vi "Sample Pad Example.vi"() -> ()   [LabVIEW 2020]
doc: "A simple sample pad, which can trigger up to 16 simultaneous sound effects. Demonstrates the Mixer component, including file loading, playback, and mixer audio monitoring via a music visualizer."
uses:
  Mixer/Channel/Controls/Channel State.ctl
  Mixer/Mixer/Mixer.lvclass/Mixer.ctl
  e8fa8eb6-c38c-4b8a-b362-922d187964a0.vi
  Mixer/Mixer/Polymorphic VIs/Channel Load (Path).vi
  Mixer/Mixer/Mixer.lvclass
  Mixer/Channel/Channel.lvclass
panel:
  in  "Labels Checkbox":bool=TRUE
  in  "Visualizer":bool
  in  "Sample Path":path
  in  "Stop":bool
  in  "Play 4":bool caption="V"
  in  "Play 3":bool caption="C"
  in  "Play 2":bool caption="X"
  in  "Play 1":bool caption="Z"
  in  "Play 8":bool caption="F"
  in  "Play 7":bool caption="D"
  in  "Play 6":bool caption="S"
  in  "Play 5":bool caption="A"
  in  "Play 12":bool caption="R"
  in  "Play 11":bool caption="E"
  in  "Play 10":bool caption="W"
  in  "Play 9":bool caption="Q"
  in  "Play 16":bool caption="4"
  in  "Play 15":bool caption="3"
  in  "Play 14":bool caption="2"
  in  "Play 13":bool caption="1"
  # "Instructions:\n1. Run the VI.\n2. Select a Sample Path which contains multiple audio files.\n3. Click a button or press the corresponding keyboard key to\n    play the audio sample.\n4. Samples can be played simultaneously, or retriggered by\n    pressing the same button / key in quick succession."
  # "G"
  # "-Audio"
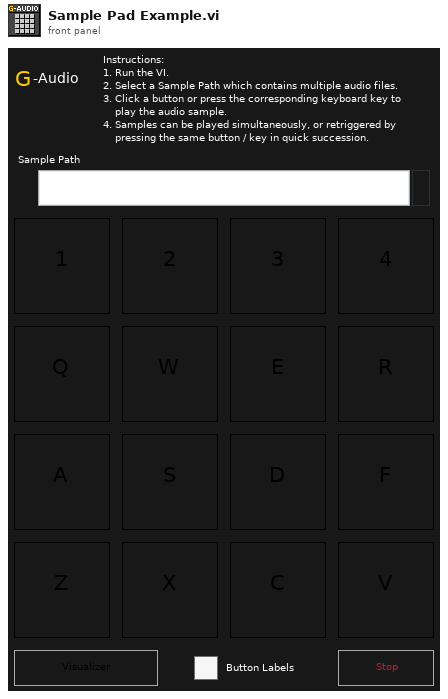
[diagram p1: front panel]
types:
  T1 = typedef "G-Audio.lvlib/Channel.lvclass/Channel State.ctl" = enum16{"Empty", "Error", "Loading", "Loaded", "Stopped", "Paused", "Playing", "Retrigger"}
  T2 = enum32{"Invalid", "Standard", "Closed", "Hidden", "Minimized", "Maximized"}
  T3 = typedef "G-Audio.lvlib/Channel.lvclass/Channel Status.ctl" = cluster{"Frame":u64, "State":T1, "Volume":dbl}
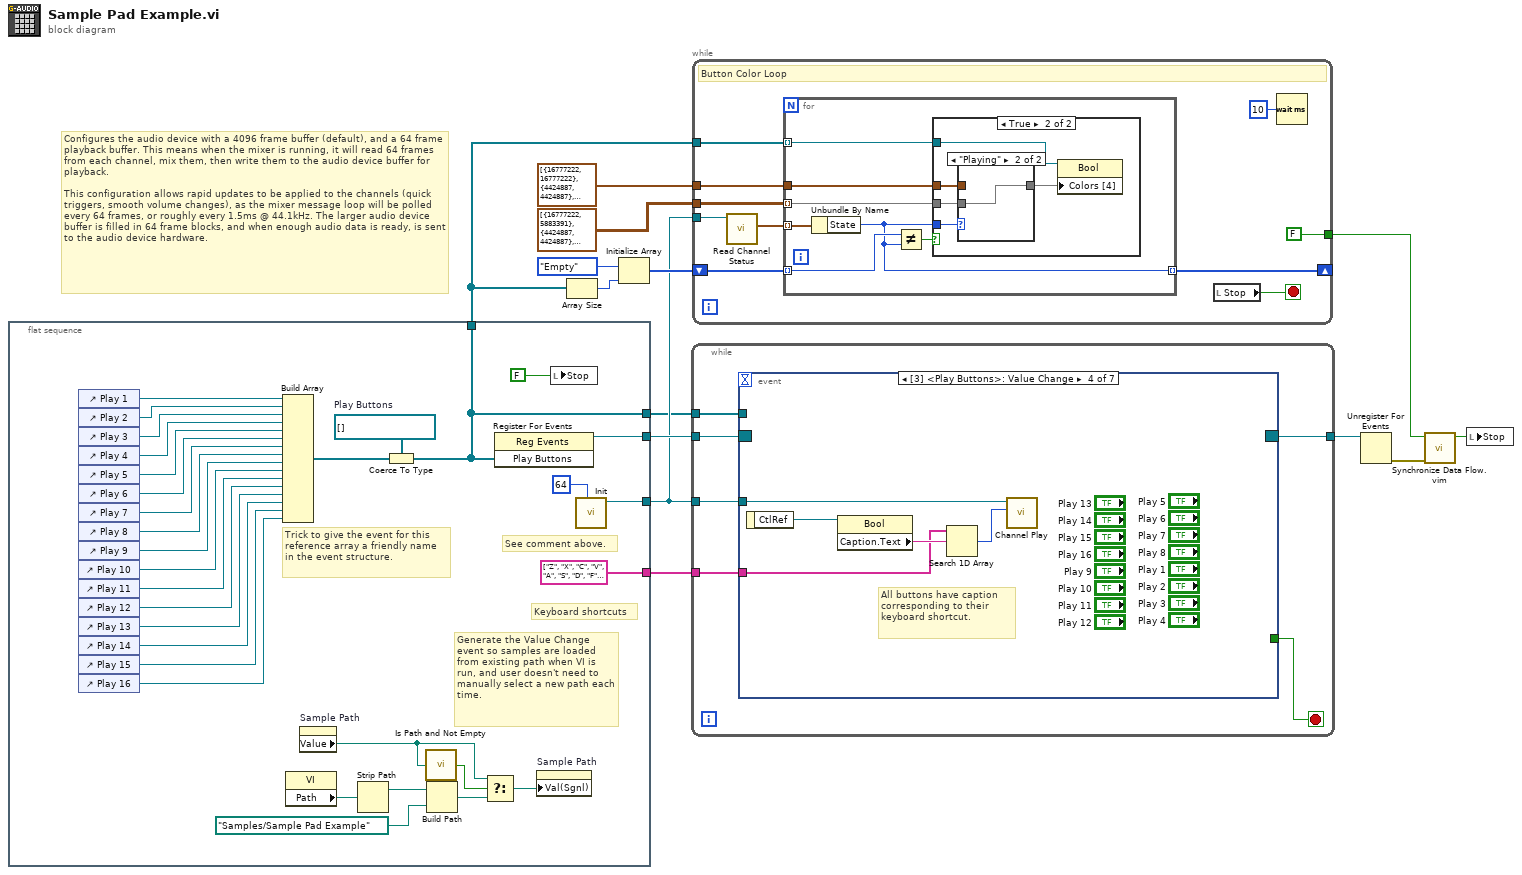
[diagram p0: block diagram]
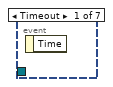
[diagram p4: hidden frame]
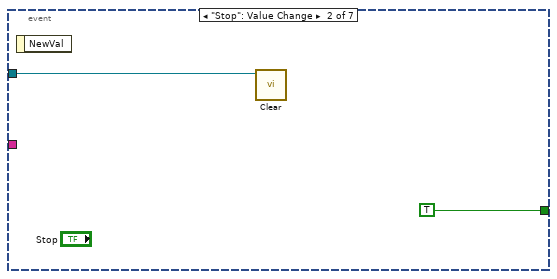
[diagram p5: hidden frame]
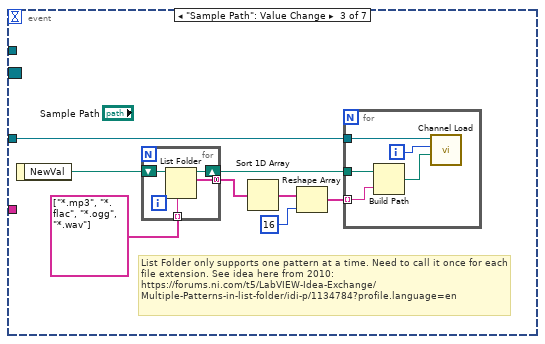
[diagram p6: hidden frame]
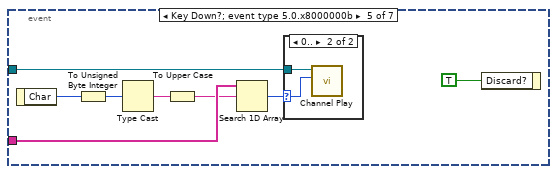
[diagram p7: hidden frame]
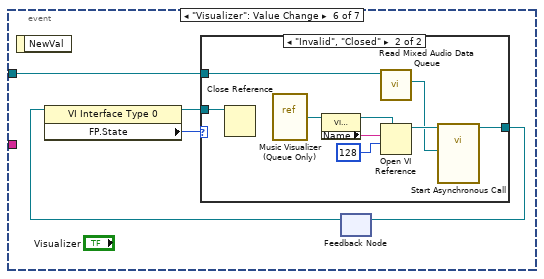
[diagram p9: hidden frame]
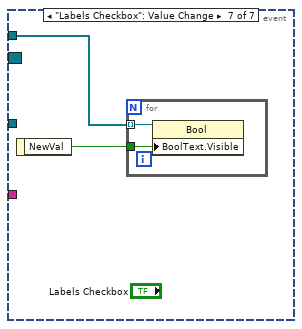
[diagram p11: hidden frame]
diagram:
  # "Configures the audio device with a 4096 frame buffer (default), and a 64 frame playback buffer. This means when the mixer is running, it will read 64 frames from each channel, mix them, then write them to the audio device buffer for playback.\n\nThis configuration allows rapid updates to be applied to the channels (quick triggers, smooth volume changes), as the mixer message loop will be polled every 64 frames, or roughly every 1.5ms @ 44.1kHz. The larger audio device buffer is filled in 64 frame blocks, and when enough audio data is ready, is sent to the audio device hardware."
  n1 = flat-sequence {
    tunnel: [w44] -> w13
    tunnel: [string[] ["Z", "X", "C", "V", "A", "S", "D", "F", "Q", "W", "E", "R", "1", "2", "3", "4"]] -> w12
    tunnel: [w15] -> w2
    tunnel: [w42] -> w5
    tunnel: [w15] -> w1
    frame #0 {
      w45 = refnum<vi>[] []  # Play Buttons
      # "Trick to give the event for this reference array a friendly name in the event structure."
      # "See comment above."
      # "Generate the Value Change event so samples are loaded from existing path when VI is run, and user doesn't need to manually select a new path each time."
      # "Keyboard shortcuts"
      n2 = control-ref of="Play 1"() -> (w39:refnum<vi>)
      n3 = control-ref of="Play 2"() -> (w38:refnum<vi>)
      n4 = control-ref of="Play 3"() -> (w37:refnum<vi>)
      n5 = control-ref of="Play 4"() -> (w36:refnum<vi>)
      n6 = control-ref of="Play 5"() -> (w35:refnum<vi>)
      n7 = control-ref of="Play 6"() -> (w34:refnum<vi>)
      n8 = control-ref of="Play 7"() -> (w33:refnum<vi>)
      n9 = control-ref of="Play 8"() -> (w32:refnum<vi>)
      n10 = control-ref of="Play 9"() -> (w31:refnum<vi>)
      n11 = control-ref of="Play 10"() -> (w30:refnum<vi>)
      n12 = control-ref of="Play 11"() -> (w29:refnum<vi>)
      n13 = control-ref of="Play 12"() -> (w28:refnum<vi>)
      n14 = control-ref of="Play 13"() -> (w27:refnum<vi>)
      n15 = control-ref of="Play 14"() -> (w26:refnum<vi>)
      n16 = control-ref of="Play 15"() -> (w25:refnum<vi>)
      n17 = control-ref of="Play 16"() -> (w24:refnum<vi>)
      n18 = Build Array(w39, w38, w37, w36, w35, w34, w33, w32, w31, w30, w29, w28, w27, w26, w25, w24) -> (w40:refnum<vi>[])
      n19 = property class="VI"() -> ("Path"=w21:path)  [unwired: 2 in, 2 out]
      n20 = property on="Sample Path" class="Path"() -> ("Value"=w17:path)  [unwired: 2 in, 2 out]
      n21 = Strip Path(path=w21) -> (stripped path=w20:path)  [unwired: 1 out]
      n22 = Coerce To Type(0:w40, 1:w45) -> (2:w15:refnum<vi>[])
      n23 = call <vilib>:"Is Path and Not Empty.vi"("path"=w17) -> ("Is Path and Not Empty?"=w23:bool)  [unwired: 4 in]
      n24 = Build Path(base path=w20, name or relative path=path "Samples/Sample Pad Example") -> (appended path=w18:path)
      n25 = Select(t=w17, s=w23, f=w18) -> (s? t:f=w22:path)
      n26 = register-events(w15) -> (reference out=w44:refnum<event-registration>)  [unwired: 2 in, 1 out]
      n27 = property on="Sample Path" class="Path"("Val(Sgnl)"=w22) -> ()  [unwired: 2 in, 2 out]
      n28 = local write "Stop"(FALSE ("Stop")) -> ()
      n29 = call "Init.vi"("Playback Size (4096)"=64) -> ("Mixer out"=w42:refnum<class "Mixer.lvclass">)  [unwired: 9 in, 1 out]
    }
  }
  n30 = Array Size(array=w2) -> (size(s)=w3:i32)
  n31 = Initialize Array(Channel_State."Empty" ("State"), w3) -> (w14:T1[])
  n32 = while {
    tunnel: w13 -> [w51]
    tunnel: w5 -> [w50]
    tunnel: w12 -> [w49]
    tunnel: [w47] -> w11
    tunnel: w1 -> [w46]
    stop <- w48 stop-if-true
    n33 = event shown="[3] <Play Buttons>: Value Change" {
      selector: w51 -> [_ _ _ _ _ _ _]
      dyn-events: [_ _ _ _ _ _ _] -> w47
      timeout: _ -> [_ _ _ _ _ _ _]
      tunnel: w50 -> [_ w53 w59 w74 w83 w89 _]
      tunnel: w49 -> [_ _ _ w72 w81 _ _]
      tunnel: [_ TRUE _ _ _ _ _] -> w48
      tunnel: w46 -> [_ _ _ _ _ _ w102]
      event Timeout {
        n34 = event-data() -> ()  [unwired: 1 in, 1 out]
      }
      event "Stop": Value Change {
        n35 = event-data() -> ()  [unwired: 1 in, 1 out]
        n36 = call "Clear.vi"("Mixer in"=w53) -> ()  [unwired: 10 in, 1 out]
      }
      event "Sample Path": Value Change {
        # "List Folder only supports one pattern at a time. Need to call it once for each file extension. See idea here from 2010:\nhttps://forums.ni.com/t5/LabVIEW-Idea-Exchange/Multiple-Patterns-in-list-folder/idi-p/1134784?profile.language=en"
        n37 = event-data() -> ("NewVal"=w54:path)  [unwired: 1 in]
        n38 = for {
          shift-right: [w65] -> w60
          shift-left: w54 -> [w64]
          tunnel: string[] ["*.mp3", "*.flac", "*.ogg", "*.wav"] -> [w63] mode=indexing
          tunnel: [w62] -> w56 mode=concatenating
          n39 = List Folder(path=w64, pattern=w63) -> (path out=w65:path, filenames=w62:string[])  [unwired: 2 in, 2 out]
        }
        n40 = Sort 1D Array(array=w56) -> (sorted array=w55:string[])
        n41 = Reshape Array(w55, 16 ("dimension size")) -> (w61:string[])
        n42 = for {
          tunnel: w61 -> [w70] mode=indexing
          tunnel: w60 -> [w69]
          tunnel: w59 -> [w68]
          i -> [w67]
          n43 = Build Path(base path=w69, name or relative path=w70) -> (appended path=w66:path)
          n44 = call-poly "Channel Load.vi"("Path"=w66, "Channel Index"=w67, "Mixer in"=w68) -> ()  [unwired: 7 in, 2 out]
        }
      }
      event Value Change {
        # "All buttons have caption corresponding to their keyboard shortcut."
        n45 = event-data() -> ("CtlRef"=w75:refnum<vi>)  [unwired: 1 in]
        n46 = property class="Bool"(reference=w75) -> ("Caption.Text"=w73:string)  [unwired: 1 in, 2 out]
        n47 = Search 1D Array(1D array=w72, element=w73) -> (index of element=w71:i32)  [unwired: 1 in]
        n48 = call "Channel Play.vi"("Channel Index"=w71, "Mixer in"=w74) -> ()  [unwired: 8 in, 2 out]
      }
      event Key Down?; event type 5.0.x8000000b {
        n49 = event-data() -> ("Char"=w82:i16)  [unwired: 1 in]
        n50 = To Unsigned Byte Integer(number=w82) -> (unsigned 8bit integer=w78:u8)
        n51 = Type Cast(x=w78) -> (*(type *) &x=w76:string)  [unwired: 1 in]
        n52 = To Upper Case(1:w76) -> (0:w79:string)
        n53 = Search 1D Array(1D array=w81, element=w79) -> (index of element=w77:i32)  [unwired: 1 in]
        n54 = case shown="0.." w77 {
          selector: w77 -> [_ w84]
          tunnel: w83 -> [_ w85]
          frame Default {
          }
          frame 0.. {
            n55 = call "Channel Play.vi"("Channel Index"=w84, "Mixer in"=w85) -> ()  [unwired: 8 in, 2 out]
          }
        }
        n56 = event-data("Discard?"=TRUE) -> ()  [unwired: 1 in, 1 out]
      }
      event "Visualizer": Value Change {
        n57 = event-data() -> ()  [unwired: 1 in, 1 out]
        n58 = feedback #1() -> (w86:refnum<vi>)  [unwired: 1 in]
        n59 = property class="VI Interface Type 0"(reference=w86) -> (reference out=w88:refnum<vi>, "FP.State"=w87:T2)  [unwired: 1 in, 1 out]
        n60 = case shown="\"Invalid\", \"Closed\"" w87 {
          tunnel: [w91 w95] -> w90
          tunnel: w89 -> [_ w94]
          tunnel: w88 -> [w91 w92]
          frame Default {
          }
          frame "Invalid", "Closed" {
            n61 = Close Reference(reference=w92) -> ()  [unwired: 1 in, 1 out]
            n62 = vi-ref "Music Visualizer (Queue Only).vi"() -> (w100:refnum<vi>)
            n63 = property class="VI (strict)"(reference=w100) -> (reference out=w98:refnum<vi>, "Name"=w99:string)  [unwired: 1 in, 1 out]
            n64 = call "Read Mixed Audio Data Queue.vi"("Mixer in"=w94) -> ("Mixed Audio Data"=w93:refnum<queue>)  [unwired: 8 in, 2 out]
            n65 = Open VI Reference(type specifier VI Refnum (for type only)=w98, vi path=w99, options=128) -> (vi reference=w96:refnum<vi>)  [unwired: 3 in, 1 out]
            n66 = call-by-ref "Start Asynchronous Call"(reference=w96, "Mixed Audio Data"=w93) -> (reference out=w95:refnum<vi>)  [unwired: 12 in, 1 out]
          }
        }
        n67 = feedback-in #1(w90) -> ()
      }
      event "Labels Checkbox": Value Change {
        n68 = event-data() -> ("NewVal"=w101:bool)  [unwired: 1 in]
        n69 = for {
          tunnel: w102 -> [w104] mode=indexing
          tunnel: w101 -> [w103]
          n70 = property class="Bool"(reference=w104, "BoolText.Visible"=w103) -> ()  [unwired: 1 in, 2 out]
        }
      }
    }
  }
  n71 = while {
    tunnel: w5 -> [w114]
    tunnel: w2 -> [w112]
    tunnel: cluster{u32, u32}[] [{16777222, 16777222}, {4424887, 4424887}, {4424887, 4424887}, {4424887, 4424887}] ("Colors [4]") -> [w111]
    tunnel: cluster{"Color Box":u32, "Color Box":u32}[][] [[{"Color Box"=16777222, "Color Box"=5883391}, {"Color Box"=4424887, "Color Box"=4424887}, {"Color Box"=4424887, "Color Box"=4424887}, {"Color Box"=4424887, "Color Box"=4424887}], [{"Color Box"=16777222, "Color Box"=5883391}, {"Color Box"=4424887, "Color Box"=4424887}, {"Color Box"=4424887, "Color Box"=4424887}, {"Color Box"=4424887, "Color Box"=4424887}], [{"Color Box"=16777222, "Color Box"=5883391}, {"Color Box"=4424887, "Color Box"=4424887}, {"Color Box"=4424887, "Color Box"=4424887}, {"Color Box"=4424887, "Color Box"=4424887}], [{"Color Box"=16777222, "Color Box"=5883391}, {"Color Box"=4424887, "Color Box"=4424887}, {"Color Box"=4424887, "Color Box"=4424887}, {"Color Box"=4424887, "Color Box"=4424887}], [{"Color Box"=16777222, "Color Box"=6618880}, {"Color Box"=4424887, "Color Box"=4424887}, {"Color Box"=4424887, "Color Box"=4424887}, {"Color Box"=4424887, "Color Box"=4424887}], [{"Color Box"=16777222, "Color Box"=6618880}, {"Color Box"=4424887, "Color Box"=4424887}, {"Color Box"=4424887, "Color Box"=4424887}, {"Color Box"=4424887, "Color Box"=4424887}], [{"Color Box"=16777222, "Color Box"=6618880}, {"Color Box"=4424887, "Color Box"=4424887}, {"Color Box"=4424887, "Color Box"=4424887}, {"Color Box"=4424887, "Color Box"=4424887}], [{"Color Box"=16777222, "Color Box"=6618880}, {"Color Box"=4424887, "Color Box"=4424887}, {"Color Box"=4424887, "Color Box"=4424887}, {"Color Box"=4424887, "Color Box"=4424887}], [{"Color Box"=16777222, "Color Box"=16746514}, {"Color Box"=4424887, "Color Box"=4424887}, {"Color Box"=4424887, "Color Box"=4424887}, {"Color Box"=4424887, "Color Box"=4424887}], [{"Color Box"=16777222, "Color Box"=16746514}, {"Color Box"=4424887, "Color Box"=4424887}, {"Color Box"=4424887, "Color Box"=4424887}, {"Color Box"=4424887, "Color Box"=4424887}], [{"Color Box"=16777222, "Color Box"=16746514}, {"Color Box"=4424887, "Color Box"=4424887}, {"Color Box"=4424887, "Color Box"=4424887}, {"Color Box"=4424887, "Color Box"=4424887}], [{"Color Box"=16777222, "Color Box"=16746514}, {"Color Box"=4424887, "Color Box"=4424887}, {"Color Box"=4424887, "Color Box"=4424887}, {"Color Box"=4424887, "Color Box"=4424887}], [{"Color Box"=16777222, "Color Box"=16711680}, {"Color Box"=4424887, "Color Box"=4424887}, {"Color Box"=4424887, "Color Box"=4424887}, {"Color Box"=4424887, "Color Box"=4424887}], [{"Color Box"=16777222, "Color Box"=16711680}, {"Color Box"=4424887, "Color Box"=4424887}, {"Color Box"=4424887, "Color Box"=4424887}, {"Color Box"=4424887, "Color Box"=4424887}], [{"Color Box"=16777222, "Color Box"=16711680}, {"Color Box"=4424887, "Color Box"=4424887}, {"Color Box"=4424887, "Color Box"=4424887}, {"Color Box"=4424887, "Color Box"=4424887}], [{"Color Box"=16777222, "Color Box"=16711680}, {"Color Box"=4424887, "Color Box"=4424887}, {"Color Box"=4424887, "Color Box"=4424887}, {"Color Box"=4424887, "Color Box"=4424887}]] ("appended array") -> [w110]
    tunnel: [FALSE ("Stop")] -> w7
    shift-right: [w106] -> _
    shift-left: w14 -> [w105]
    stop <- w108 stop-if-true
    # "Button Color Loop"
    n72 = call "Read Channel Status.vi"("Mixer in"=w114) -> ("Channel Status"=w113:T3[])  [unwired: 8 in, 2 out]
    n73 = for {
      tunnel: w113 -> [w121] mode=indexing
      tunnel: w112 -> [w120] mode=indexing
      tunnel: w111 -> [w119]
      tunnel: w110 -> [w118] mode=indexing
      tunnel: [w115] -> w106 mode=indexing
      tunnel: w105 -> [w117] mode=indexing
      n74 = Unbundle By Name(w121) -> ("State"=w115:T1)
      n75 = Not Equal?(x=w117, y=w115) -> (x != y?=w116:bool)
      n76 = case shown="True" w116 {
        tunnel: w120 -> [_ w126]
        tunnel: w119 -> [_ w125]
        tunnel: w118 -> [_ w123]
        tunnel: w115 -> [_ w122]
        frame False {
        }
        frame True {
          n77 = case shown="\"Playing\"" w122 {
            tunnel: w125 -> [w127 _]
            tunnel: [w127 w128] -> w124
            tunnel: w123 -> [_ w128]
            frame Default {
            }
            frame "Playing" {
            }
          }
          n78 = property class="Bool"(reference=w126, "Colors [4]"=w124) -> ()  [unwired: 1 in, 2 out]
        }
      }
    }
    n79 = local read "Stop"() -> (w108:bool)
    n80 = Wait (ms)(milliseconds to wait=u32 10) -> ()  [unwired: 1 out]
  }
  n81 = Unregister For Events(event registration refnum=w11) -> (error out=w8:errorcluster)  [unwired: 1 in]
  n82 = call "Synchronize Data Flow.vim"("input 4"=w8, "input 1"=w7) -> ("output 1"=w9:bool)  [unwired: 2 in, 3 out]
  n83 = local write "Stop"(w9) -> ()
